vi "Drive Immediate.vi"(6 "Throttle Setpoint":dbl, 7 "Description":string, 8 "Command Info In":T1, 9 "Deadband Value":dbl=0.01, 10 "Right Setpoint":dbl, 11 "Left Setpoint":dbl) -> (0 "Command Info Out":T1)   [LabVIEW 2015]
doc: "Often used for joystick control, this VI checks to see that the joystick axes are outside the deadband and updates the motors appropriately."
uses:
  <vilib>/Rock Robotics/WPI/Framework/Command Status Info.ctl
  <vilib>/Rock Robotics/WPI/Framework/Completion Status.ctl
  <vilib>/Rock Robotics/WPI/Framework/Completion Notifier.ctl
  Implementation/Drive Setpoints.ctl
  Implementation/Drive Operations.ctl
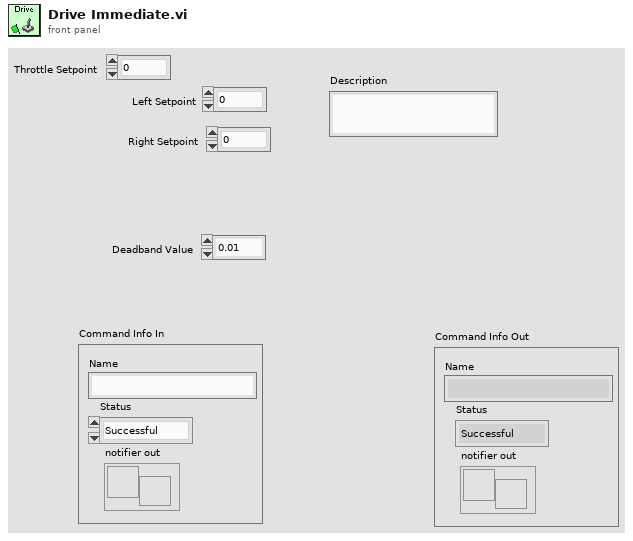
[diagram p1: front panel]
types:
  T1 = typedef "Command Status Info.ctl" = cluster{"Name":string, "Status":T2, "notifier out":T3}
  T2 = typedef "Completion Status.ctl" = enum16{"Successful", "Aborted", "Incomplete"}
  T3 = typedef "Completion Notifier.ctl" = refnum<notifier>
  T4 = typedef "Drive Setpoints.ctl" = cluster{"Operation":T5, "Left Setpoint":dbl, "Right Setpoint":dbl, "Duration":dbl, "Throttle Setpoint":dbl}
  T5 = typedef "Drive Operations.ctl" = enum16{"Reserve", "Read Current", "Immediate", "Drive for Time", "Drive for Distance"}
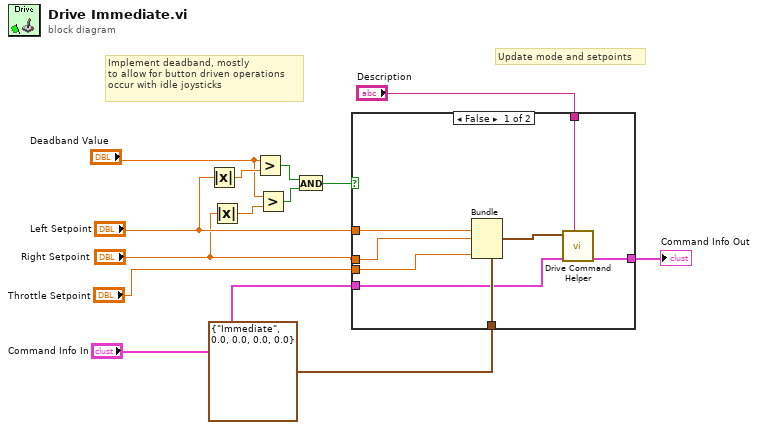
[diagram p0: block diagram]
diagram:
  # "Implement deadband, mostly\nto allow for button driven operations\noccur with idle joysticks"
  # "Update mode and setpoints"
  n1 = Absolute Value(x="Left Setpoint") -> (abs(x)=w13:dbl)
  n2 = Absolute Value(x="Right Setpoint") -> (abs(x)=w5:dbl)
  n3 = Greater?(x="Deadband Value", y=w13) -> (0:w7:bool)
  n4 = Greater?(x="Deadband Value", y=w5) -> (0:w3:bool)
  n5 = And(x=w7, y=w3) -> (x .and. y?=w6:bool)
  n6 = case shown="False" w6 {
    tunnel: "Left Setpoint" -> [w21 _]
    tunnel: T4 {"Operation"=enum."Immediate", "Left Setpoint"=0.0, "Right Setpoint"=0.0, "Duration"=0.0, "Throttle Setpoint"=0.0} ("SubSystem Data") -> [w20 _]
    tunnel: [w19 w22] -> w12
    tunnel: "Command Info In" -> [w18 w22]
    tunnel: "Description" -> [w16 _]
    tunnel: "Right Setpoint" -> [w15 _]
    tunnel: "Throttle Setpoint" -> [w14 _]
    frame False {
      n7 = Bundle(cluster=w20, "Left Setpoint"=w21, "Right Setpoint"=w15, "Throttle Setpoint"=w14) -> (w17:T4)  [unwired: 2 in]
      n8 = call "Drive Command Helper.vi"("Description"=w16, "Command Info In"=w18, "SubSystem Data"=w17) -> ("Command Info Out"=w19:T1)  [unwired: 7 in, 1 out]
    }
    frame True {
    }
  }
  "Command Info Out" <- w12
